vi "IMURead.vi"(0 "AdaIMUDevRef":T4={"DevStatus"={"status"=FALSE, "code"=0, "source"=""}, "Gyro Address"=0, "Gyro Range"=0, "Mean Rates"={"Xmo"=0.0, "Ymo"=0.0, "Zmo"=0.0}, "StdDev Rates"={"Xsdo"=0.0, "Ysdo"=0.0, "Zsdo"=0.0}, "Fast"=FALSE, "Reset"=FALSE, "Accel Address"=0, "Accel Range"=0, "Accel Scale"={"Xscale"=0.0, "Yscale"=0.0, "Zscale"=0.0}, "Mag Address"=0, "Mag Range"=0, "G Sense"=FALSE, "A Sense"=FALSE, "M Sense"=FALSE, "Accel Offset"={"Xzero"=0.0, "Yzero"=0.0, "Zzero"=0.0}, "Motion Thresh"=0.0, "Mag Scale"={"Xscale"=1.0, "Yscale"=1.0, "Zscale"=1.0}, "Mag Offset"={"Xzero"=1.0, "Yzero"=1.0, "Zzero"=1.0}, "I2C Bus"=enum."I2C On-Board", "Handle"=0, "Controller"=enum."Controller 1", "Anomaly Thresh"=0.0, "Local Mag"=0.0}, 11 "error in":errorcluster) -> (4 "AdaIMUDevRef Out":T4={"DevStatus"={"status"=FALSE, "code"=0, "source"=""}, "Gyro Address"=0, "Gyro Range"=0, "Mean Rates"={"Xmo"=0.0, "Ymo"=0.0, "Zmo"=0.0}, "StdDev Rates"={"Xsdo"=0.0, "Ysdo"=0.0, "Zsdo"=0.0}, "Fast"=FALSE, "Reset"=FALSE, "Accel Address"=0, "Accel Range"=0, "Accel Scale"={"Xscale"=0.0, "Yscale"=0.0, "Zscale"=0.0}, "Mag Address"=0, "Mag Range"=0, "G Sense"=FALSE, "A Sense"=FALSE, "M Sense"=FALSE, "Accel Offset"={"Xzero"=0.0, "Yzero"=0.0, "Zzero"=0.0}, "Motion Thresh"=0.0, "Mag Scale"={"Xscale"=1.0, "Yscale"=1.0, "Zscale"=1.0}, "Mag Offset"={"Xzero"=1.0, "Yzero"=1.0, "Zzero"=1.0}, "I2C Bus"=enum."I2C On-Board", "Handle"=0, "Controller"=enum."Controller 1", "Anomaly Thresh"=0.0, "Local Mag"=0.0}, 6 "Gyro":T3, 8 "Accel":T1={"Xaccel"=0.0, "Yaccel"=0.0, "Zaccel"=0.0, "Motion"=FALSE, "Threshold"=0.04, "FreeFall"=FALSE}, 10 "Mag":T2, 15 "error out":errorcluster)   [LabVIEW 2014]
uses:
  IMUDevRef.ctl
  <vilib>/Rock Robotics/SystemInterfaces/i2clib/i2c_bus.ctl
  <vilib>/Rock Robotics/SystemInterfaces/Typedef/FPGA_TypedefDigitalModule.ctl
  Gyro.ctl
  Mag.ctl
  Accel.ctl
  <vilib>/Rock Robotics/WPI/I2C/WPI_I2CDevRef.ctl
panel:
  # "When Sensor oriented with positive X-axis\npointing forward, and positive Y-axis\npointing left, and positive Z axis pointing up :\n\nRoll is rotation about X-axis, clockwise roll,\n(looking in + X direction), is positive.\n\nPitch is rotation about Y-axis, clockwise pitch\n(looking in + Y direction), is positive.\n\nYaw is rotation about Z-axis, clockwise yaw\n(looking in + Z direction), is positive."
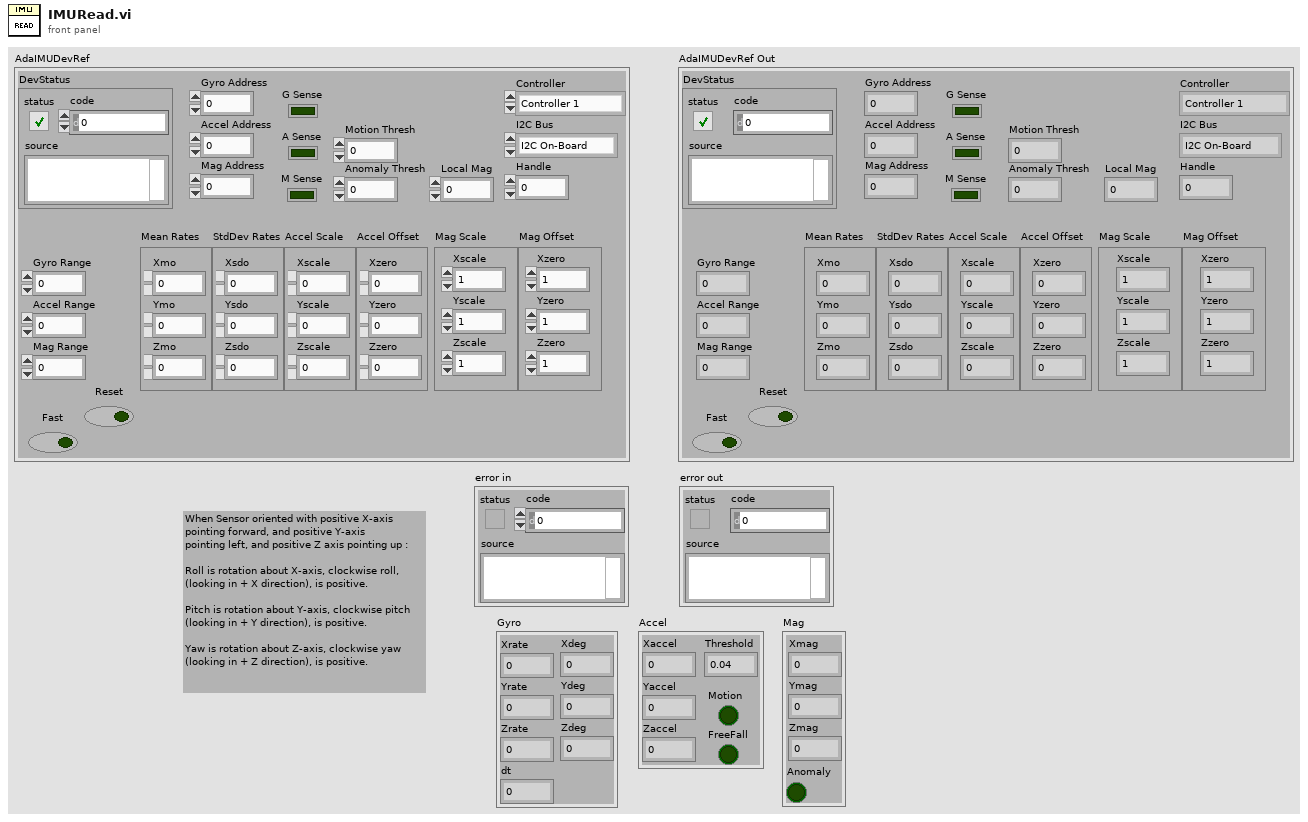
[diagram p1: front panel]
types:
  T1 = typedef "Accel.ctl" = cluster{"Xaccel":dbl, "Yaccel":dbl, "Zaccel":dbl, "Motion":bool, "Threshold":dbl, "FreeFall":bool}
  T2 = typedef "Mag.ctl" = cluster{"Xmag":dbl, "Ymag":dbl, "Zmag":dbl, "Anomaly":bool}
  T3 = typedef "Gyro.ctl" = cluster{"Xrate":dbl, "Yrate":dbl, "Zrate":dbl, "Xdeg":dbl, "Ydeg":dbl, "Zdeg":dbl, "dt":dbl}
  T4 = typedef "IMUDevRef.ctl" = cluster{"DevStatus":errorcluster, "Gyro Address":u8, "Gyro Range":u8, "Mean Rates":cluster{"Xmo":dbl, "Ymo":dbl, "Zmo":dbl}, "StdDev Rates":cluster{"Xsdo":dbl, "Ysdo":dbl, "Zsdo":dbl}, "Fast":bool, "Reset":bool, "Accel Address":u8, "Accel Range":u8, "Accel Scale":cluster{"Xscale":dbl, "Yscale":dbl, "Zscale":dbl}, "Mag Address":u8, "Mag Range":u8, "G Sense":bool, "A Sense":bool, "M Sense":bool, "Accel Offset":cluster{"Xzero":dbl, "Yzero":dbl, "Zzero":dbl}, "Motion Thresh":dbl, "Mag Scale":cluster{"Xscale":dbl, "Yscale":dbl, "Zscale":dbl}, "Mag Offset":cluster{"Xzero":dbl, "Yzero":dbl, "Zzero":dbl}, "I2C Bus":T5, "Handle":i32, "Controller":T6, "Anomaly Thresh":dbl, "Local Mag":dbl}
  T5 = typedef "i2c_bus.ctl" = enum16{"I2C On-Board", "I2C MXP", "Invalid"}
  T6 = typedef "FPGA_TypedefDigitalModule.ctl" = enum16{"Controller 1"}
  T7 = typedef "WPI_I2CDevRef.ctl" = cluster{"DevStatus":errorcluster, "Controller":T6, "Device Address":u8, "Handle":i32, "I2C Bus":T5}
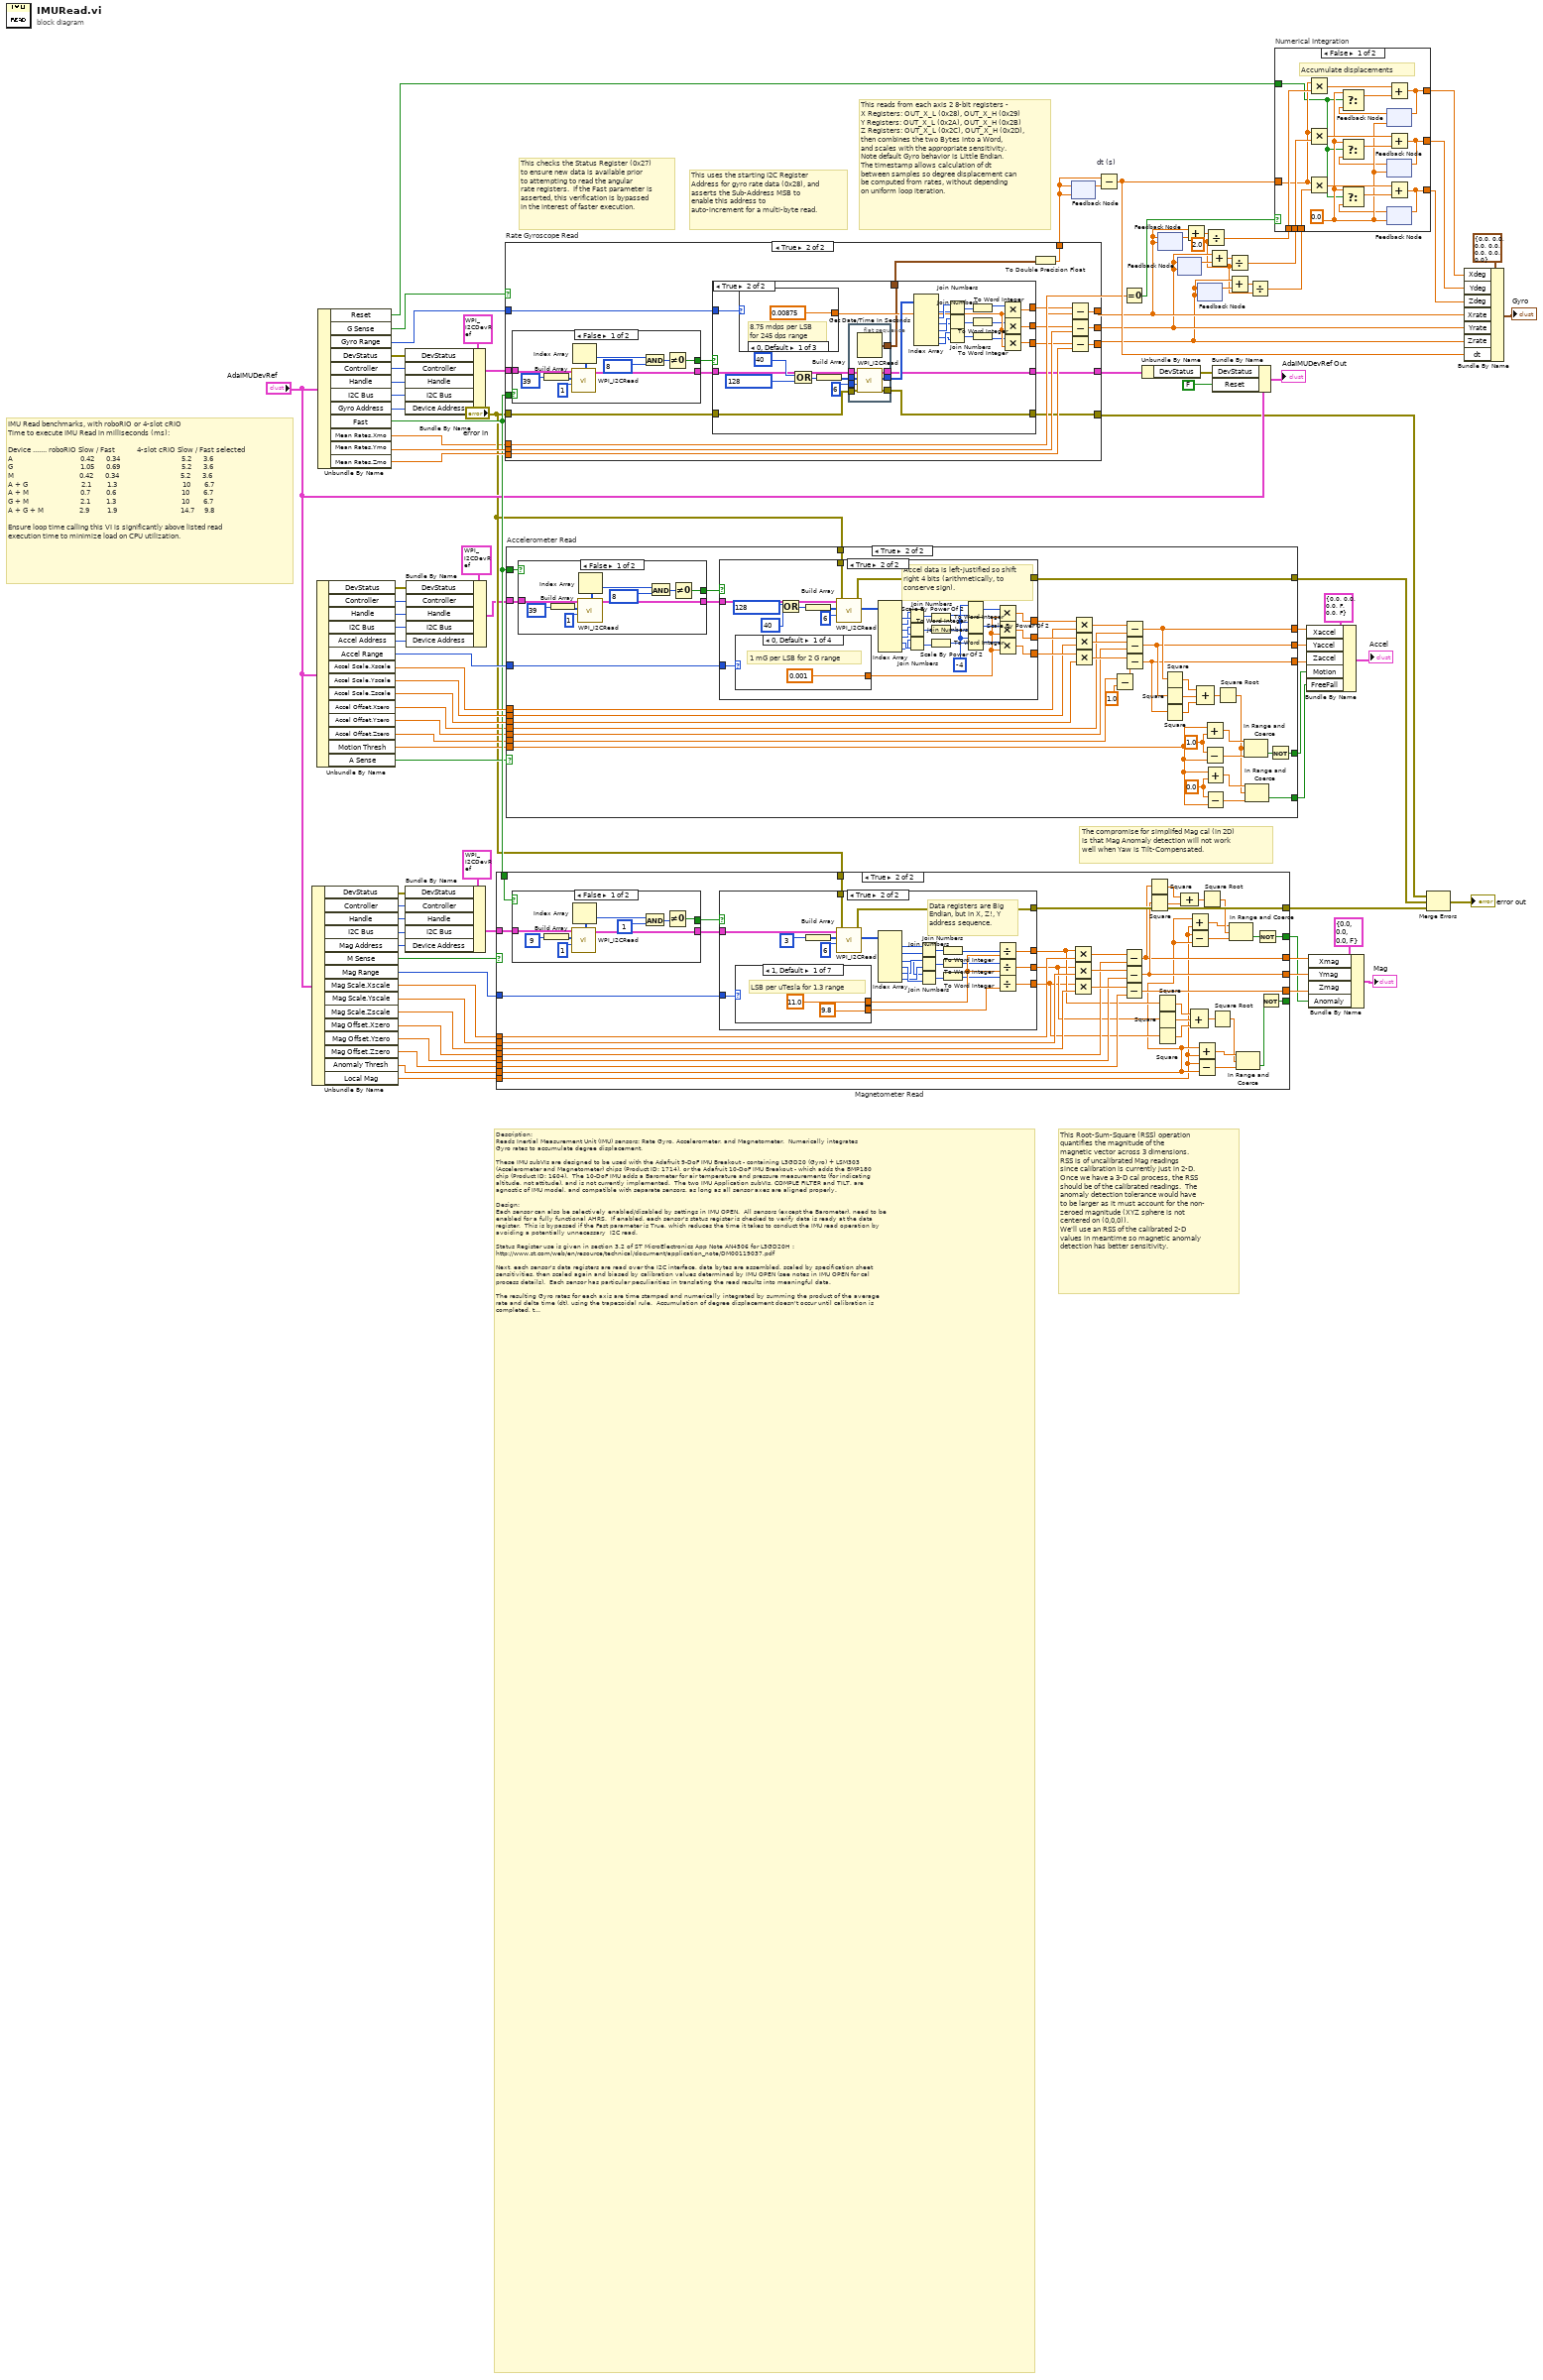
[diagram p0: block diagram]
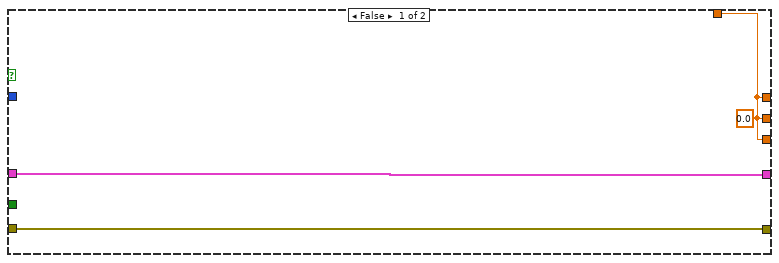
[diagram p2: hidden frame]
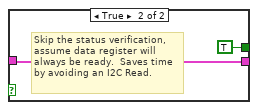
[diagram p3: hidden frame]
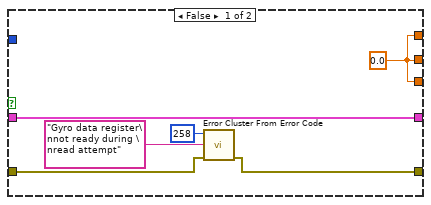
[diagram p4: hidden frame]
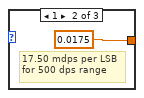
[diagram p5: hidden frame]
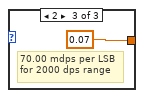
[diagram p6: hidden frame]
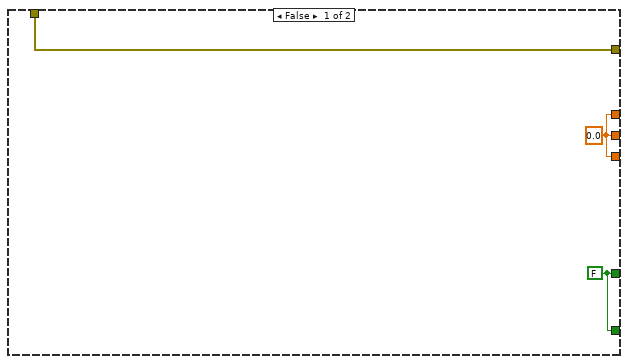
[diagram p7: hidden frame]
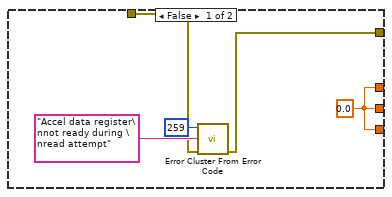
[diagram p8: hidden frame]
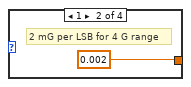
[diagram p9: hidden frame]
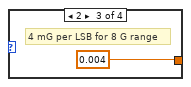
[diagram p10: hidden frame]
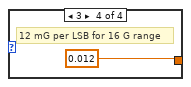
[diagram p11: hidden frame]
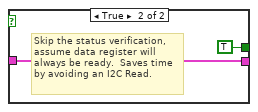
[diagram p12: hidden frame]
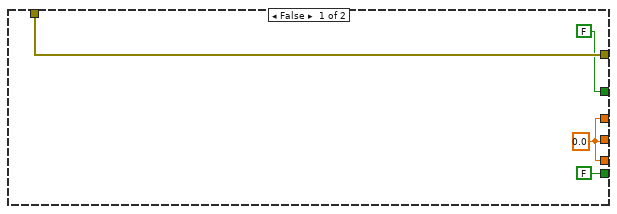
[diagram p13: hidden frame]
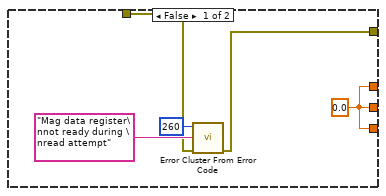
[diagram p14: hidden frame]
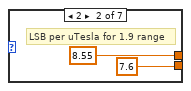
[diagram p15: hidden frame]
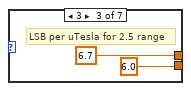
[diagram p16: hidden frame]
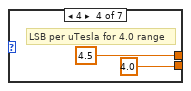
[diagram p17: hidden frame]
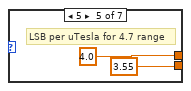
[diagram p18: hidden frame]
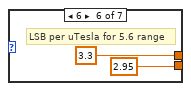
[diagram p19: hidden frame]
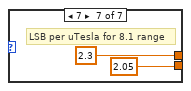
[diagram p20: hidden frame]
diagram:
  w22 = 2.0 ("y")
  # "The compromise for simplifed Mag cal (in 2D)\nis that Mag Anomaly detection will not work\nwell when Yaw is Tilt-Compensated."
  # "This Root-Sum-Square (RSS) operation\nquantifies the magnitude of the\nmagnetic vector across 3 dimensions.\nRSS is of uncalibrated Mag readings\nsince calibration is currently just in 2-D.\nOnce we have a 3-D cal process, the RSS\nshould be of the calibrated readings.  The\nanomaly detection tolerance would have \nto be larger as it must account for the non-\nzeroed magnitude (XYZ sphere is not\ncentered on (0,0,0)). \nWe'll use an RSS of the calibrated 2-D\nvalues in meantime so magnetic anomaly\ndetection has better sensitivity."
  # "Description:\nReads Inertial Measurement Unit (IMU) sensors: Rate Gyro, Accelerometer, and Magnetometer.  Numerically integrates\nGyro rates to accumulate degree displacement.\n\nThese IMU subVIs are designed to be used with the Adafruit 9-DoF IMU Breakout - containing L3GD20 (Gyro) + LSM303 \n(Accelerometer and Magnetometer) chips (Product ID: 1714), or the Adafruit 10-DoF IMU Breakout - which adds the BMP180\nchip (Product ID: 1604).  The 10-DoF IMU adds a Barometer for air temperature and pressure measurements (for indicating\naltitude, not attitude), and is not currently implemented.  The two IMU Application subVIs, COMPLE FILTER and TILT, are\nagnostic of IMU model, and compatible with separate sensors, as long as all sensor axes are aligned properly.\n\nDesign:\nEach sensor can also be selectively enabled/disabled by settings in IMU OPEN.  All sensors (except the Barometer), need to be\nenabled for a fully functional AHRS.  If enabled, each sensor's status register is checked to verify data is ready at the data\nregister.  This is bypassed if the Fast parameter is True, which reduces the time it takes to conduct the IMU read operation by\navoiding a potentially unnecessary  I2C read.  \n\nStatus Register use is given in section 3.2 of ST MicroElectronics App Note AN4506 for L3GD20H : \nhttp://www.st.com/web/en/resource/technical/document/application_note/DM00119037.pdf\n\nNext, each sensor's data registers are read over the I2C interface, data bytes are assembled, scaled by specification sheet\nsensitivities, then scaled again and biased by calibration values determined by IMU OPEN (see notes in IMU OPEN for cal\nprocess details).  Each sensor has particular peculiarities in translating the read results into meaningful data.\n\nThe resulting Gyro rates for each axis are time stamped and numerically integrated by summing the product of the average\nrate and delta time (dt), using the trapezoidal rule.  Accumulation of degree displacement doesn't occur until calibration is\ncompleted, to allow IMU OPEN to make use of IMU READ for the cal process (code reuse).  Resetting the degree displacements\nto zero is accomplished by IMU RESET generating a flag via the IMU DevRef cluster, requiring the 'reset' signal to always be\nupstream of the IMU READ, which is then cleared here.  The native data register sequence is Little Endian - review this term and\nits relationship to Gulliver’s Travels by Jonathan Swift for insight on reference.  Rates, Degrees, and dt are provided in a Gyro\noutput cluster.\n\nAlthough each sensor shares the basic design of storing their measurements across two one-byte registers, the Accelerometer\ndata registers are left-justified (and Little Endian), with the lowest 4 bits of the lowest byte containing no data.  (Gyro and\nMagnetometer data registers are both right-justified.)  Presumably the left-justification provides a means to read the Accel\nfaster by reading only the upper byte, should one not require the additional precision contained in the lower byte.  Since we\nare using both bytes for maximum precision, the concatenation of the two bytes must be right-shifted by 4 bits.  This must be\ndone with an arithmetic shift, rather than a logical shift, to preserve the sign bit encoded within the twos-complement storage\nformat.  \n\nMovement and Free Fall are detected by comparing the root-sum-square of the 3 axes to value 1 (G) for movement\ndetection and 0 (G) for Free Fall using a common Threshold value as tolerance for the comparison.  A future improvement is to\ntake advantage of the Accelerometer's on-board Free Fall detection capability, i.e., moving the detection into hardware for\nsuperior response, which could be sensed with a DIO port. Each calibrated axis reading is provided in a Accel output cluster\nalong with Movement and Free Fall Booleans.\n\nThe Magnetometer data registers are Big Endian, but are peculiar in that the register address sequence is X-Z-Y instead of X-Y-Z.\nThis is non-obvious and was clearly done to simply torture me.  Magnetic Anomalies are detected by comparing the\nroot-sum-square of the X and Y axes (2-D) to the horizontal magnitude of the local Earth field.  One can use the value calculated\nduring the magnetic calibration process, which should be consistent with data available at the National Geophysical Data Center\n\n(NOAA/NGDC at http://www.ngdc.noaa.gov/geomag-web/?useFullSite=true#igrfwmm)\n\n... input USA zip code or city/country, select Get Lat/Long then Calculate, and note \"Horizontal Intensity\", expressing this in\nmicroTeslas (not nanoTeslas as NOAA displays).  An Anomaly Threshold value is used as tolerance for the comparison.  Each\ncalibrated axis reading is provided in a Mag output cluster along with a Magnetic Anomaly Boolean.\n\nInputs:\nADAIMUDEVREF - Device Reference containing IMU configuration data.  Sensor enable condition, range, I2C address, and\n                                calibration parameters are stored here.\nOutputs:\nADAIMUDEVREF OUT - Device Reference containing IMU configuration data.  Gyro reset is cleared as each IMU READ completes.\nGYRO - Cluster containing rate and displacements for each axis with delta time since last data point.\nACCEL - Cluster containing, for each axis, calibrated acceleration measurement with movement/free fall indications and threshold.\nMAG - Cluster containing, for each axis, calibrated magnetic measurement with magnetic anomaly indication.\nANOMALY - Boolean indicating that a magnetic anomaly is detected.\n\nFuture Improvements:\nMove freefall into interrupt/DIO, Auto ranging, FPGA numerical integration or Simpson's Rule to improve off-FPGA numerical\nintegration, SPI interface for potentially faster read response.\n\n\nVI Properties:\nExecution Reentrancy is set to Non Reentrant Execution\n\nImplementation:\nThis design performs numerical integration off-FPGA for the Digital Gyro (unlike the Analog Gyro subVIs, which typically utilize\nthe FPGA to perform accumulation for superior speed resulting in less integration error).   Testing indicates this off-FPGA\napproach may be adequate for FRC application, however, it is important to ensure the code runs without any timing issues.\nThis is why a Timed Loop is recommended for the IMU Read within Periodic Tasks (executes at a higher priority).  Non-uniformity\nin read iteration is mitigated by design, as each dt is uniquely calculated by time stamping each read event.  This means that while\nsome variation in timing can be tolerated (the occasional late iteration), excessively long durations (periods) between successive\nreads will fail to capture the actual rate profile as it changes resulting in integration error.  \n\nIn short, use a Timed Loop structure to iterate IMU READs, and set the loop period for a relatively fast iteration (<75 ms).  Shorter\nperiods provide improved accuracy of degree displacements, however setting this too short can impact the execution of your\nremaining code (especially when using Timed Loops).  One way of determining an optimized period is to set it while monitoring\nthe \"Finished Late?\" Loop parameter, ensuring this value stays False.   It helps if the CPU Utilization remains low (<75%), which\ncan be monitored with the RT Get CPU Loads subVI (Real Time menu).  Study LabVIEW determinism for additional insight.\n\nIMU Read benchmarks, with roboRIO or 4-slot cRIO\nTime to execute IMU Read in milliseconds (ms):\n\nSensor ....... roboRIO Slow / Fast           4-slot cRIO Slow / Fast selected\nA                                  0.42      0.34                               5.2      3.6\nG                                  1.05      0.69                               5.2      3.6\nM                                 0.42      0.34                               5.2      3.6\nA + G                           2.1        1.3                                 10       6.7\nA + M                          0.7        0.6                                 10       6.7\nG + M                          2.1        1.3                                 10       6.7\nA + G + M                  2.9         1.9                                14.7     9.8\n\n(\"Slow\" is when Fast is deasserted).\n\nEnsure loop time calling this VI is significantly above listed read execution time to minimize load on CPU utilization.\n\n----- The RoboBees FRC Team 836! -----  You too can conquer inertia!! ... consider a career in STEM!"
  # "IMU Read benchmarks, with roboRIO or 4-slot cRIO\nTime to execute IMU Read in milliseconds (ms):\n\nDevice ....... roboRIO Slow / Fast           4-slot cRIO Slow / Fast selected\nA                                  0.42      0.34                               5.2      3.6\nG                                  1.05      0.69                               5.2      3.6\nM                                 0.42      0.34                               5.2      3.6\nA + G                           2.1        1.3                                 10       6.7\nA + M                          0.7        0.6                                 10       6.7\nG + M                          2.1        1.3                                 10       6.7\nA + G + M                  2.9         1.9                                14.7     9.8\n\nEnsure loop time calling this VI is significantly above listed read\nexecution time to minimize load on CPU utilization."
  # "This reads from each axis 2 8-bit registers - \nX Registers: OUT_X_L (0x28), OUT_X_H (0x29)\nY Registers: OUT_X_L (0x2A), OUT_X_H (0x2B)\nZ Registers: OUT_X_L (0x2C), OUT_X_H (0x2D),\nthen combines the two Bytes into a Word,\nand scales with the appropriate sensitivity.\nNote default Gyro behavior is Little Endian.\nThe timestamp allows calculation of dt\nbetween samples so degree displacement can\nbe computed from rates, without depending\non uniform loop iteration."
  # "This checks the Status Register (0x27)\nto ensure new data is available prior\nto attempting to read the angular\nrate registers.  If the Fast parameter is\nasserted, this verification is bypassed\nin the interest of faster execution."
  # "This uses the starting I2C Register\nAddress for gyro rate data (0x28), and\nasserts the Sub-Address MSB to\nenable this address to \nauto-increment for a multi-byte read."
  n1 = Unbundle By Name("AdaIMUDevRef") -> ("DevStatus"=w66:errorcluster, "Controller"=w67:T6, "Handle"=w11:i32, "I2C Bus"=w10:T5, "Mag Address"=w12:u8, "M Sense"=w48:bool, "Mag Range"=w49:u8, "Mag Scale.Xscale"=w8:dbl, "Mag Scale.Yscale"=w33:dbl, "Mag Scale.Zscale"=w36:dbl, "Mag Offset.Xzero"=w35:dbl, "Mag Offset.Yzero"=w34:dbl, "Mag Offset.Zzero"=w9:dbl, "Anomaly Thresh"=w7:dbl, "Local Mag"=w6:dbl)
  n2 = Unbundle By Name("AdaIMUDevRef") -> ("DevStatus"=w76:errorcluster, "Controller"=w75:T6, "Handle"=w13:i32, "I2C Bus"=w14:T5, "Accel Address"=w15:u8, "Accel Range"=w74:u8, "Accel Scale.Xscale"=w73:dbl, "Accel Scale.Yscale"=w72:dbl, "Accel Scale.Zscale"=w71:dbl, "Accel Offset.Xzero"=w58:dbl, "Accel Offset.Yzero"=w57:dbl, "Accel Offset.Zzero"=w56:dbl, "Motion Thresh"=w50:dbl, "A Sense"=w47:bool)
  n3 = Unbundle By Name("AdaIMUDevRef") -> ("Reset"=w44:bool, "G Sense"=w43:bool, "Gyro Range"=w70:u8, "DevStatus"=w78:errorcluster, "Controller"=w79:T6, "Handle"=w18:i32, "I2C Bus"=w17:T5, "Gyro Address"=w16:u8, "Fast"=w65:bool, "Mean Rates.Xmo"=w19:dbl, "Mean Rates.Ymo"=w91:dbl, "Mean Rates.Zmo"=w92:dbl)
  n4 = Bundle By Name(cluster=T7 {"DevStatus"={"status"=FALSE, "code"=0, "source"=""}, "Controller"=enum."Controller 1", "Device Address"=107, "Handle"=28, "I2C Bus"=enum."I2C On-Board"} ("I2CDevRef 2"), "DevStatus"=w78, "Controller"=w79, "Handle"=w18, "I2C Bus"=w17, "Device Address"=w16) -> (w69:T7)
  n5 = Bundle By Name(cluster=T7 {"DevStatus"={"status"=FALSE, "code"=0, "source"=""}, "Controller"=enum."Controller 1", "Device Address"=107, "Handle"=28, "I2C Bus"=enum."I2C On-Board"} ("I2CDevRef 2"), "DevStatus"=w66, "Controller"=w67, "Handle"=w11, "I2C Bus"=w10, "Device Address"=w12) -> (w68:T7)
  n6 = Bundle By Name(cluster=T7 {"DevStatus"={"status"=FALSE, "code"=0, "source"=""}, "Controller"=enum."Controller 1", "Device Address"=107, "Handle"=28, "I2C Bus"=enum."I2C On-Board"} ("I2CDevRef 2"), "DevStatus"=w76, "Controller"=w75, "Handle"=w13, "I2C Bus"=w14, "Device Address"=w15) -> (w5:T7)
  n7 = case "Magnetometer Read" shown="True" w48 {
    tunnel: w68 -> [_ w137]
    tunnel: w49 -> [_ w134]
    tunnel: "error in" -> [w95 w133]
    tunnel: [w95 w132] -> w38
    tunnel: w65 -> [_ w131]
    tunnel: [w96 w100] -> w62
    tunnel: [w96 w101] -> w61
    tunnel: [w96 w115] -> w60
    tunnel: w8 -> [_ w127]
    tunnel: w33 -> [_ w126]
    tunnel: w36 -> [_ w125]
    tunnel: w35 -> [_ w124]
    tunnel: w34 -> [_ w123]
    tunnel: w9 -> [_ w122]
    tunnel: [FALSE w110] -> _
    tunnel: w7 -> [_ w99]
    tunnel: w6 -> [_ w98]
    tunnel: [FALSE w97] -> w1
    frame False {
      w96 = 0.0
    }
    frame True {
      n8 = case shown="False" w131 {
        tunnel: w137 -> [w182 w192]
        tunnel: [w187 w192] -> w135
        tunnel: [w183 TRUE] -> w136
        frame False {
          n9 = Build Array(u8 9 ("Data To Send")) -> (w191:u8[])
          n10 = call <vilib>:"WPI_I2CRead.vi"("I2CBytesToRead"=u8 1, "I2CRegister"=w191, "I2CDevRef"=w182) -> ("Data Out"=w188:u8[], "I2CDevRef"=w187:T7)  [unwired: 6 in, 1 out]
          n11 = Index Array(array=w188) -> (element=w185:u8)  [unwired: 1 in]
          n12 = And(x=w185, y=u8 1 ("Data To Send")) -> (x .and. y?=w184:u8)
          n13 = Not Equal To 0?(x=w184) -> (x != 0?=w183:bool)
        }
        frame True {
          # "Skip the status verification,\nassume data register will\nalways be ready.  Saves time\nby avoiding an I2C Read."
        }
      }
      n14 = case shown="True" w136 {
        tunnel: [w142 w160] -> w113
        tunnel: [w142 w159] -> w112
        tunnel: [w142 w158] -> w111
        tunnel: w134 -> [_ w157]
        tunnel: w135 -> [_ w156]
        tunnel: w133 -> [w139 w155]
        tunnel: [w138 w154] -> w132
        frame False {
          w142 = 0.0
          n15 = call <vilib>:"Error Cluster From Error Code.vi"("error in (no error)"=w139, "error message (\"\")"="Mag data register\nnot ready during \nread attempt" ("error message (\"\")"), "error code (0)"=260) -> ("error out"=w138:errorcluster)  [unwired: 6 in]
        }
        frame True {
          # "Data registers are Big\nEndian, but in X, Z!, Y\naddress sequence."
          n16 = case shown="1, Default" w157 {
            tunnel: [11.0 ("y") 8.55 ("y") 6.7 ("y") 4.5 ("y") 4.0 ("y") 3.3 ("y") 2.3 ("y")] -> w161
            tunnel: [9.8 ("y") 7.6 ("y") 6.0 ("y") 4.0 ("y") 3.55 ("y") 2.95 ("y") 2.05 ("y")] -> w147
            frame 1, Default {
              # "LSB per uTesla for 1.3 range"
            }
            frame 2 {
              # "LSB per uTesla for 1.9 range"
            }
            frame 3 {
              # "LSB per uTesla for 2.5 range"
            }
            frame 4 {
              # "LSB per uTesla for 4.0 range"
            }
            frame 5 {
              # "LSB per uTesla for 4.7 range"
            }
            frame 6 {
              # "LSB per uTesla for 5.6 range"
            }
            frame 7 {
              # "LSB per uTesla for 8.1 range"
            }
          }
          n17 = Build Array(u8 3 ("Data To Send")) -> (w164:u8[])
          n18 = call <vilib>:"WPI_I2CRead.vi"("error in (no error)"=w155, "I2CBytesToRead"=u8 6, "I2CRegister"=w164, "I2CDevRef"=w156) -> ("error out"=w154:errorcluster, "Data Out"=w166:u8[])  [unwired: 5 in, 1 out]
          n19 = Index Array(array=w166) -> (element #1=w152:u8, element #2=w151:u8, element #3=w143:u8, element #4=w146:u8, element #5=w145:u8, element #6=w144:u8)  [unwired: 6 in]
          n20 = Join Numbers(hi=w152, lo=w151) -> ((hi.lo)=w165:u16)
          n21 = Join Numbers(hi=w145, lo=w144) -> ((hi.lo)=w162:u16)
          n22 = Join Numbers(hi=w143, lo=w146) -> ((hi.lo)=w163:u16)
          n23 = To Word Integer(number=w165) -> (16bit integer=w150:i16)
          n24 = To Word Integer(number=w162) -> (16bit integer=w149:i16)
          n25 = To Word Integer(number=w163) -> (16bit integer=w148:i16)
          n26 = Divide(x=w150, y=w161) -> (x/y=w160:dbl)
          n27 = Divide(x=w149, y=w161) -> (x/y=w159:dbl)
          n28 = Divide(x=w148, y=w147) -> (x/y=w158:dbl)
        }
      }
      n29 = Multiply(x=w113, y=w127) -> (x*y=w128:dbl)
      n30 = Multiply(x=w112, y=w126) -> (x*y=w129:dbl)
      n31 = Multiply(x=w111, y=w125) -> (x*y=w130:dbl)
      n32 = Subtract(x=w128, y=w124) -> (x-y=w100:dbl)
      n33 = Subtract(x=w129, y=w123) -> (x-y=w101:dbl)
      n34 = Subtract(x=w130, y=w122) -> (x-y=w115:dbl)
      n35 = Square(x=w100) -> (x^2=w106:dbl)
      n36 = Square(x=w101) -> (x^2=w105:dbl)
      n37 = Square(x=w113) -> (x^2=w116:dbl)
      n38 = Square(x=w112) -> (x^2=w117:dbl)
      n39 = Square(x=w111) -> (x^2=w118:dbl)
      n40 = Compound Arithmetic op=ADD(w106, w105) -> (w104:dbl)
      n41 = Add(x=w99, y=w98) -> (x+y=w102:dbl)
      n42 = Subtract(x=w98, y=w99) -> (x-y=w103:dbl)
      n43 = Compound Arithmetic op=ADD(w116, w117, w118) -> (w119:dbl)
      n44 = Add(x=w99, y=w98) -> (x+y=w121:dbl)
      n45 = Subtract(x=w98, y=w99) -> (x-y=w120:dbl)
      n46 = Square Root(x=w104) -> (sqrt(x)=w107:dbl)
      n47 = Square Root(x=w119) -> (sqrt(x)=w114:dbl)
      n48 = In Range and Coerce(upper limit=w102, x=w107, lower limit=w103) -> (In Range?=w108:bool)  [unwired: 1 out]
      n49 = In Range and Coerce(upper limit=w121, x=w114, lower limit=w120) -> (In Range?=w109:bool)  [unwired: 1 out]
      n50 = Not(x=w108) -> (.not. x?=w97:bool)
      n51 = Not(x=w109) -> (.not. x?=w110:bool)
    }
  }
  n52 = case "Rate Gyroscope Read" shown="True" w43 {
    tunnel: w92 -> [_ w215]
    tunnel: w91 -> [_ w214]
    tunnel: w19 -> [_ w213]
    tunnel: [w196 w209] -> w23
    tunnel: [w196 w207] -> w81
    tunnel: w70 -> [_ w204]
    tunnel: w69 -> [w195 w203]
    tunnel: [w194 w202] -> w42
    tunnel: w65 -> [_ w201]
    tunnel: [w196 w200] -> w29
    tunnel: [w196 w199] -> w24
    tunnel: [w195 w198] -> w46
    tunnel: "error in" -> [w194 w197]
    frame False {
      w196 = 0.0
    }
    frame True {
      n53 = case shown="False" w201 {
        tunnel: w203 -> [w216 w227]
        tunnel: [w221 w227] -> w206
        tunnel: [w218 TRUE] -> w205
        frame False {
          n54 = Build Array(u8 39 ("Data To Send")) -> (w225:u8[])
          n55 = call <vilib>:"WPI_I2CRead.vi"("I2CBytesToRead"=u8 1, "I2CRegister"=w225, "I2CDevRef"=w216) -> ("Data Out"=w222:u8[], "I2CDevRef"=w221:T7)  [unwired: 6 in, 1 out]
          n56 = Index Array(array=w222) -> (element=w219:u8)  [unwired: 1 in]
          n57 = And(x=w219, y=u8 8 ("Data To Send")) -> (x .and. y?=w220:u8)
          n58 = Not Equal To 0?(x=w220) -> (x != 0?=w218:bool)
        }
        frame True {
          # "Skip the status verification,\nassume data register will\nalways be ready.  Saves time\nby avoiding an I2C Read."
        }
      }
      n59 = case shown="True" w205 {
        tunnel: [w229 w261] -> w212
        tunnel: w197 -> [w233 w260]
        tunnel: [w232 w259] -> w202
        tunnel: w206 -> [w228 w250]
        tunnel: [w229 w247] -> w211
        tunnel: [w229 w246] -> w210
        tunnel: w204 -> [_ w243]
        tunnel: [_ w241] -> w208
        tunnel: [w228 w234] -> w198
        frame False {
          w229 = 0.0
          n60 = call <vilib>:"Error Cluster From Error Code.vi"("error in (no error)"=w233, "error message (\"\")"="Gyro data register\nnot ready during \nread attempt" ("error message (\"\")"), "error code (0)"=258) -> ("error out"=w232:errorcluster)  [unwired: 6 in]
        }
        frame True {
          n61 = case shown="0, Default" w243 {
            tunnel: [0.00875 ("y") 0.0175 ("y") 0.07 ("y")] -> w242
            frame 0, Default {
              # "8.75 mdps per LSB\nfor 245 dps range"
            }
            frame 1 {
              # "17.50 mdps per LSB\nfor 500 dps range"
            }
            frame 2 {
              # "70.00 mdps per LSB\nfor 2000 dps range"
            }
          }
          n62 = Or(x=u8 40 ("Data To Send"), y=u8 128 ("Data To Send")) -> (x .or. y?=w255:u8)
          n63 = Build Array(w255) -> (w257:u8[])
          n64 = flat-sequence {
            tunnel: w260 -> [w269]
            tunnel: [w268] -> w259
            tunnel: [w267] -> w258
            tunnel: w257 -> [w266]
            tunnel: u8 6 ("I2CBytesToRead") -> [w265]
            tunnel: w250 -> [w264]
            tunnel: [w263] -> w241
            tunnel: [w262] -> w234
            frame #0 {
              n65 = Get Date/Time In Seconds() -> (seconds since 1Jan1904=w263:timestamp)
              n66 = call <vilib>:"WPI_I2CRead.vi"("error in (no error)"=w269, "I2CBytesToRead"=w265, "I2CRegister"=w266, "I2CDevRef"=w264) -> ("error out"=w268:errorcluster, "Data Out"=w267:u8[], "I2CDevRef"=w262:T7)  [unwired: 5 in]
            }
          }
          n67 = Index Array(array=w258) -> (element #1=w251:u8, element #2=w252:u8, element #3=w244:u8, element #4=w245:u8, element #5=w248:u8, element #6=w249:u8)  [unwired: 6 in]
          n68 = Join Numbers(hi=w252, lo=w251) -> ((hi.lo)=w240:u16)
          n69 = Join Numbers(hi=w245, lo=w244) -> ((hi.lo)=w238:u16)
          n70 = Join Numbers(hi=w249, lo=w248) -> ((hi.lo)=w237:u16)
          n71 = To Word Integer(number=w240) -> (16bit integer=w239:i16)
          n72 = To Word Integer(number=w238) -> (16bit integer=w236:i16)
          n73 = To Word Integer(number=w237) -> (16bit integer=w235:i16)
          n74 = Multiply(x=w239, y=w242) -> (x*y=w261:dbl)
          n75 = Multiply(x=w236, y=w242) -> (x*y=w247:dbl)
          n76 = Multiply(x=w235, y=w242) -> (x*y=w246:dbl)
        }
      }
      n77 = To Double Precision Float(number=w208) -> (double precision float=w207:dbl)
      n78 = Subtract(x=w212, y=w213) -> (x-y=w200:dbl)
      n79 = Subtract(x=w211, y=w214) -> (x-y=w199:dbl)
      n80 = Subtract(x=w210, y=w215) -> (x-y=w209:dbl)
    }
  }
  n81 = case "Accelerometer Read" shown="True" w47 {
    tunnel: w74 -> [_ w311]
    tunnel: w73 -> [_ w310]
    tunnel: w72 -> [_ w309]
    tunnel: w71 -> [_ w308]
    tunnel: w5 -> [_ w305]
    tunnel: [w274 w304] -> w39
    tunnel: "error in" -> [w274 w303]
    tunnel: w65 -> [_ w302]
    tunnel: w58 -> [_ w298]
    tunnel: w57 -> [_ w297]
    tunnel: w56 -> [_ w295]
    tunnel: [w275 w293] -> w55
    tunnel: [w275 w292] -> w54
    tunnel: [w275 w291] -> w53
    tunnel: [w273 w282] -> w51
    tunnel: w50 -> [_ w278]
    tunnel: [w273 w277] -> w37
    frame False {
      w275 = 0.0
      w273 = FALSE
    }
    frame True {
      w280 = 0.0 ("upper limit")
      w285 = 1.0 ("upper limit")
      n82 = case shown="False" w302 {
        tunnel: w305 -> [w354 w364]
        tunnel: [w358 w364] -> w307
        tunnel: [w355 TRUE] -> w306
        frame False {
          n83 = Build Array(u8 39 ("Data To Send")) -> (w362:u8[])
          n84 = call <vilib>:"WPI_I2CRead.vi"("I2CBytesToRead"=u8 1, "I2CRegister"=w362, "I2CDevRef"=w354) -> ("Data Out"=w359:u8[], "I2CDevRef"=w358:T7)  [unwired: 6 in, 1 out]
          n85 = Index Array(array=w359) -> (element=w357:u8)  [unwired: 1 in]
          n86 = And(x=w357, y=u8 8 ("Data To Send")) -> (x .and. y?=w356:u8)
          n87 = Not Equal To 0?(x=w356) -> (x != 0?=w355:bool)
        }
        frame True {
          # "Skip the status verification,\nassume data register will\nalways be ready.  Saves time\nby avoiding an I2C Read."
        }
      }
      n88 = case shown="True" w306 {
        tunnel: [w319 w330] -> w314
        tunnel: [w319 w329] -> w313
        tunnel: [w319 w328] -> w312
        tunnel: w311 -> [_ w327]
        tunnel: w307 -> [_ w326]
        tunnel: w303 -> [w316 w325]
        tunnel: [w315 w324] -> w304
        frame False {
          w319 = 0.0
          n89 = call <vilib>:"Error Cluster From Error Code.vi"("error in (no error)"=w316, "error message (\"\")"="Accel data register\nnot ready during \nread attempt" ("error message (\"\")"), "error code (0)"=259) -> ("error out"=w315:errorcluster)  [unwired: 6 in]
        }
        frame True {
          w320 = i16 -4 ("y")
          # "Accel data is left-justified so shift right 4 bits (arithmetically, to conserve sign)."
          n90 = case shown="0, Default" w327 {
            tunnel: [0.001 ("y") 0.002 ("y") 0.004 ("y") 0.012 ("y")] -> w331
            frame 0, Default {
              # "1 mG per LSB for 2 G range"
            }
            frame 1 {
              # "2 mG per LSB for 4 G range"
            }
            frame 2 {
              # "4 mG per LSB for 8 G range"
            }
            frame 3 {
              # "12 mG per LSB for 16 G range"
            }
          }
          n91 = Or(x=u8 128 ("Data To Send"), y=u8 40 ("Data To Send")) -> (x .or. y?=w344:u8)
          n92 = Build Array(w344) -> (w343:u8[])
          n93 = call <vilib>:"WPI_I2CRead.vi"("error in (no error)"=w325, "I2CBytesToRead"=u8 6, "I2CRegister"=w343, "I2CDevRef"=w326) -> ("error out"=w324:errorcluster, "Data Out"=w348:u8[])  [unwired: 5 in, 1 out]
          n94 = Index Array(array=w348) -> (element #1=w346:u8, element #2=w342:u8, element #3=w339:u8, element #4=w338:u8, element #5=w337:u8, element #6=w336:u8)  [unwired: 6 in]
          n95 = Join Numbers(hi=w342, lo=w346) -> ((hi.lo)=w347:u16)
          n96 = Join Numbers(hi=w338, lo=w339) -> ((hi.lo)=w340:u16)
          n97 = Join Numbers(hi=w336, lo=w337) -> ((hi.lo)=w341:u16)
          n98 = To Word Integer(number=w347) -> (16bit integer=w322:i16)
          n99 = To Word Integer(number=w340) -> (16bit integer=w323:i16)
          n100 = To Word Integer(number=w341) -> (16bit integer=w321:i16)
          n101 = Scale By Power Of 2(n=w320, x=w322) -> (x*2^n=w332:i16)
          n102 = Scale By Power Of 2(n=w320, x=w323) -> (x*2^n=w334:i16)
          n103 = Scale By Power Of 2(n=w320, x=w321) -> (x*2^n=w333:i16)
          n104 = Multiply(x=w332, y=w331) -> (x*y=w330:dbl)
          n105 = Multiply(x=w334, y=w331) -> (x*y=w329:dbl)
          n106 = Multiply(x=w333, y=w331) -> (x*y=w328:dbl)
        }
      }
      n107 = Multiply(x=w314, y=w310) -> (x*y=w301:dbl)
      n108 = Multiply(x=w313, y=w309) -> (x*y=w300:dbl)
      n109 = Multiply(x=w312, y=w308) -> (x*y=w299:dbl)
      n110 = Subtract(x=w295, y=1.0 ("x")) -> (x-y=w296:dbl)
      n111 = Subtract(x=w301, y=w298) -> (x-y=w293:dbl)
      n112 = Subtract(x=w300, y=w297) -> (x-y=w292:dbl)
      n113 = Subtract(x=w299, y=w296) -> (x-y=w291:dbl)
      n114 = Square(x=w293) -> (x^2=w290:dbl)
      n115 = Square(x=w292) -> (x^2=w289:dbl)
      n116 = Square(x=w291) -> (x^2=w288:dbl)
      n117 = Compound Arithmetic op=ADD(w290, w289, w288) -> (w287:dbl)
      n118 = Add(x=w278, y=w285) -> (x+y=w286:dbl)
      n119 = Subtract(x=w285, y=w278) -> (x-y=w284:dbl)
      n120 = Add(x=w278, y=w280) -> (x+y=w279:dbl)
      n121 = Subtract(x=w280, y=w278) -> (x-y=w281:dbl)
      n122 = Square Root(x=w287) -> (sqrt(x)=w276:dbl)
      n123 = In Range and Coerce(upper limit=w286, x=w276, lower limit=w284) -> (In Range?=w283:bool)  [unwired: 1 out]
      n124 = In Range and Coerce(upper limit=w279, x=w276, lower limit=w281) -> (In Range?=w277:bool)  [unwired: 1 out]
      n125 = Not(x=w283) -> (.not. x?=w282:bool)
    }
  }
  n126 = feedback #1(w81) -> (w82:dbl)
  n127 = feedback-in #1(w81) -> ()
  n128 = Subtract "dt (s)"(x=w81, y=w82) -> (x-y=w59:dbl)
  n129 = Equal To 0?(x=w19) -> (x = 0?=w86:bool)
  n130 = Unbundle By Name(w46) -> ("DevStatus"=w90:errorcluster)
  n131 = feedback #2(w29) -> (w32:dbl)
  n132 = feedback-in #2(w29) -> ()
  n133 = feedback #3(w24) -> (w27:dbl)
  n134 = feedback-in #3(w24) -> ()
  n135 = Add(x=w29, y=w32) -> (x+y=w31:dbl)
  n136 = feedback #4(w23) -> (w26:dbl)
  n137 = feedback-in #4(w23) -> ()
  n138 = Divide(x=w31, y=w22) -> (x/y=w30:dbl)
  n139 = Add(x=w24, y=w27) -> (x+y=w28:dbl)
  n140 = Bundle By Name(cluster="AdaIMUDevRef", "DevStatus"=w90, "Reset"=FALSE ("Fast")) -> (→"AdaIMUDevRef Out":T4)
  n141 = Divide(x=w28, y=w22) -> (x/y=w21:dbl)
  n142 = Add(x=w23, y=w26) -> (x+y=w25:dbl)
  n143 = Divide(x=w25, y=w22) -> (x/y=w20:dbl)
  n144 = case "Numerical Integration" shown="False" w86 {
    tunnel: w20 -> [w383 _]
    tunnel: [w382 w384] -> w85
    tunnel: w59 -> [w376 _]
    tunnel: w21 -> [w381 _]
    tunnel: w30 -> [w379 _]
    tunnel: [w378 w384] -> w84
    tunnel: [w377 w384] -> w83
    tunnel: w44 -> [w366 _]
    frame False {
      w369 = 0.0
      # "Accumulate displacements"
      n145 = Multiply(x=w376, y=w379) -> (x*y=w380:dbl)
      n146 = Multiply(x=w376, y=w381) -> (x*y=w373:dbl)
      n147 = Multiply(x=w376, y=w383) -> (x*y=w372:dbl)
      n148 = feedback #5(w369) -> (w374:dbl)
      n149 = Select(t=w369, s=w366, f=w374) -> (s? t:f=w375:dbl)
      n150 = Add(x=w380, y=w375) -> (x+y=w377:dbl)
      n151 = feedback-in #5(w377) -> ()
      n152 = feedback #6(w369) -> (w368:dbl)
      n153 = Select(t=w369, s=w366, f=w368) -> (s? t:f=w371:dbl)
      n154 = Add(x=w373, y=w371) -> (x+y=w378:dbl)
      n155 = feedback-in #6(w378) -> ()
      n156 = feedback #7(w369) -> (w367:dbl)
      n157 = Select(t=w369, s=w366, f=w367) -> (s? t:f=w370:dbl)
      n158 = Add(x=w372, y=w370) -> (x+y=w382:dbl)
      n159 = feedback-in #7(w382) -> ()
    }
    frame True {
      w384 = 0.0
      # "Avoid accumulating\ndegree displacements\nuntil calibrated\n(Once zero rate offsets\nare non-zero)."
    }
  }
  n160 = Bundle By Name(cluster=T1 {"Xaccel"=0.0, "Yaccel"=0.0, "Zaccel"=0.0, "Motion"=FALSE, "Threshold"=0.0, "FreeFall"=FALSE} ("input cluster"), "Xaccel"=w55, "Yaccel"=w54, "Zaccel"=w53, "Motion"=w51, "FreeFall"=w37) -> (→"Accel":T1)
  n161 = Bundle By Name(cluster=T2 {"Xmag"=0.0, "Ymag"=0.0, "Zmag"=0.0, "Anomaly"=FALSE}, "Xmag"=w62, "Ymag"=w61, "Zmag"=w60, "Anomaly"=w1) -> (→"Mag":T2)
  n162 = Merge Errors(w42, w39, w38) -> (→"error out":errorcluster)
  n163 = Bundle By Name(cluster=T3 {"Xrate"=0.0, "Yrate"=0.0, "Zrate"=0.0, "Xdeg"=0.0, "Ydeg"=0.0, "Zdeg"=0.0, "dt"=0.0} ("input cluster"), "Xdeg"=w83, "Ydeg"=w84, "Zdeg"=w85, "Xrate"=w29, "Yrate"=w24, "Zrate"=w23, "dt"=w59) -> (→"Gyro":T3)
